vi "DLTS - setup impedance (SubVI).vi"(0 "Handle Out in":T1 {"Handle" format="0x%08x"; "Conn" format="0x%08x"}, 1 "IMPS current range":dbl, 3 "IMPS output range":dbl=10.0 format="%#_13g", 5 "IMPS test signal":dbl, 7 "Output on":bool=TRUE, 9 "IMPS test freq":dbl, 11 "error in (no error)":errorcluster, 12 "IMPS  bandwidth":dbl=5000.0, 13 "IMPS auto bandwidth control":bool=TRUE, 14 "IMPS demod sampling rate":dbl) -> (4 "Handle Out out":T1 {"Handle" format="0x%08x"; "Conn" format="0x%08x"}, 15 "error out":errorcluster)   [LabVIEW 2019]
doc: "Configures impedance analyzer settings for a DLTS measurement"
uses:
  <instrlib>/Zurich Instruments LabOne/Public/ziTypeHandle.ctl
  <instrlib>/Zurich Instruments LabOne/Public/Configure/ziSetValueDoubleArray.vi
  <instrlib>/Zurich Instruments LabOne/Zurich Instruments LabOne.lvlib
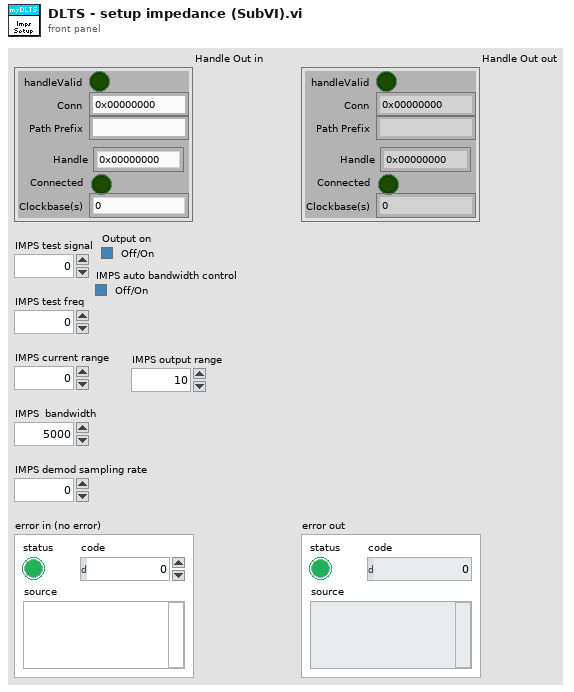
[diagram p1: front panel]
types:
  T1 = typedef "Zurich Instruments LabOne.lvlib/ziTypeHandle.ctl" = cluster{"handleValid":bool, "Conn":u64, "Path Prefix":string, "Handle":u64, "Connected":bool, "Clockbase(s)":dbl}
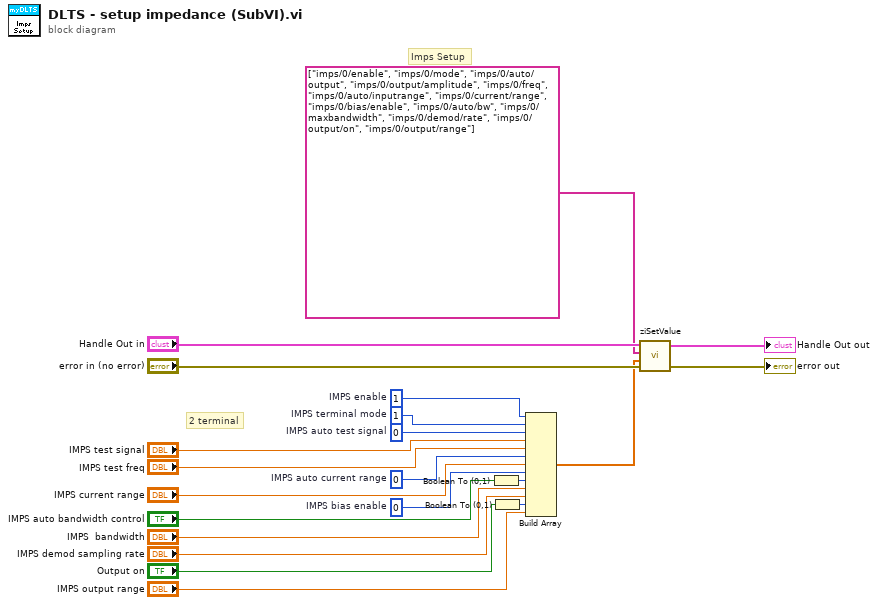
[diagram p0: block diagram]
diagram:
  w1 = 0  # IMPS auto current range
  w15 = 1  # IMPS terminal mode
  w10 = 0  # IMPS bias enable
  w7 = 0  # IMPS auto test signal
  w14 = 1  # IMPS enable
  # "2 terminal"
  # "Imps Setup"
  n1 = Boolean To (0,1)(Boolean="IMPS auto bandwidth control") -> (0, 1=w3:i16)
  n2 = Boolean To (0,1)(Boolean="Output on") -> (0, 1=w6:i16)
  n3 = Build Array(w14, w15, w7, "IMPS test signal", "IMPS test freq", w1, "IMPS current range", w10, w3, "IMPS  bandwidth", "IMPS demod sampling rate", w6, "IMPS output range") -> (w12:dbl[])
  n4 = call-poly <instrlib>:"ziSetValue.vi"("Error In"="error in (no error)", "Values"=w12, "Paths"=string[] ["imps/0/enable", "imps/0/mode", "imps/0/auto/output", "imps/0/output/amplitude", "imps/0/freq", "imps/0/auto/inputrange", "imps/0/current/range", "imps/0/bias/enable", "imps/0/auto/bw", "imps/0/maxbandwidth", "imps/0/demod/rate", "imps/0/output/on", "imps/0/output/range"], "Handle In"="Handle Out in") -> ("Error Out"=→"error out":errorcluster, "Handle Out"=→"Handle Out out":T1)  [unwired: 1 in]
